vi "playerase.vi"() -> ()   [LabVIEW 2014]
panel:
  in  "stop":bool
  in  "input":bool
  out "num 2":dbl
  out "num 1":dbl
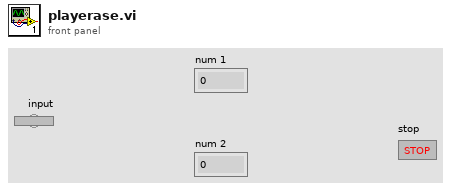
[diagram p1: front panel]
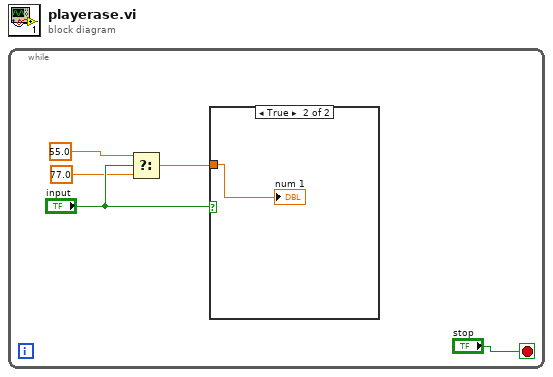
[diagram p0: block diagram]
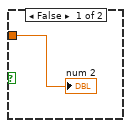
[diagram p2: hidden frame]
diagram:
  n1 = while {
    stop <- "stop" stop-if-true
    n2 = Select(t=55.0, s="input", f=77.0) -> (s? t:f=w1:dbl)
    n3 = case shown="True" "input" {
      tunnel: w1 -> [w6 w7]
      frame False {
        "num 2" <- w6
      }
      frame True {
        "num 1" <- w7
      }
    }
  }
